vi "merFISH_init_ramp_brightfield.vi"(2 "error in":errorcluster, 3 "Piezo queue":refnum<queue>) -> (0 "error out":errorcluster, 1 "Piezo queue out":refnum<queue>)   [LabVIEW 2015]
uses:
  CONTROLS/Q_MCL_piezo_element.ctl
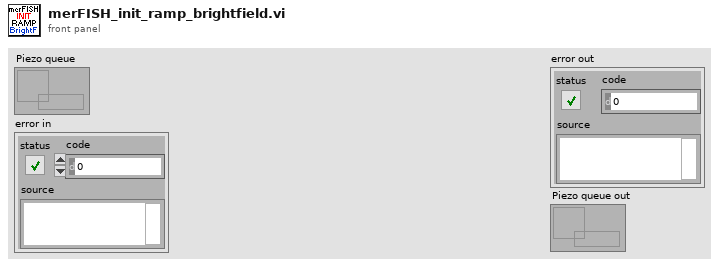
[diagram p1: front panel]
types:
  T1 = typedef "Q_MCL_piezo_element.ctl" = cluster{"variant":variant, "Instruction":enum16{"Piezo_idle", "Piezo_initialize", "Piezo_error", "Piezo_security_stop", "Piezo_read_z", "Piezo_move_z", "Piezo_keyboard_move", "Piezo_close_autofocus_calibration_ramp", "Piezo_change_init_state", "Piezo_init_autofocus", "Piezo_init_autofocus_merFISH_TL", "Piezo_autofocus", "Piezo_autofocus_merFISH_TL", "Piezo_stop_autofocus", "Piezo_stop_autofocus_merFISH_TL", "Piezo_autofocus_lost", "Piezo_resume_autofocus_merFISH_TL", "Piezo_check_z_position_merFISH_TL", "Piezo_init_ramp", "Piezo_move_z_ramp", "Piezo_close_ramp", "Piezo_close_merFISH", "Piezo_stop"}}
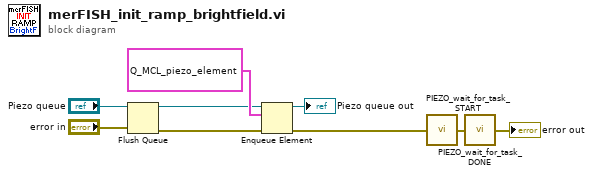
[diagram p0: block diagram]
diagram:
  n1 = Flush Queue(queue="Piezo queue", error in (no error)="error in") -> (queue out=w6:refnum<queue>, error out=w5:errorcluster)  [unwired: 1 out]
  n2 = Enqueue Element(queue=w6, element=T1 {"variant"=variant, "Instruction"=enum."Piezo_init_ramp"} ("Q_MCL_Piezo"), error in (no error)=w5) -> (queue out=→"Piezo queue out":refnum<queue>, error out=w9:errorcluster)  [unwired: 1 in, 1 out]
  n3 = call "PIEZO_wait_for_task_START.vi"("error in"=w9) -> ("error out"=w8:errorcluster)
  n4 = call "PIEZO_wait_for_task_DONE.vi"("error in"=w8) -> ("error out"=→"error out":errorcluster)
